vi "Write Scheduled.vi"(1 "scheduled time":timestamp, 2 "element":bool) -> (5 "actual time":timestamp, 7 "channel":T1, 8 "previous element":bool)   [LabVIEW 2020, in "Tag-bool.lvlib"]
doc: "Writes a value to a Tag channel at the scheduled time."
uses:
  <extravilib>/ChannelInstances/Tag-bool.lvlib
  <extravilib>/ChannelInstances/Tag-bool/))Channel.ctl
  <extravilib>/ChannelInstances/Tag-bool/Write With Abort.vi
  <extravilib>/ChannelInstances/Tag-bool/Endpoint.vi
  <resource>/ChannelSupport/_ChannelSupport/_ChannelSupport.lvlib
  <resource>/ChannelSupport/_ChannelSupport/GetErrors/FpgaChannelWireNotSupported.xnode
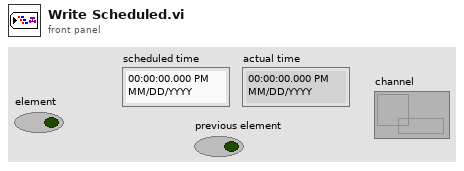
[diagram p1: front panel]
types:
  T1 = typedef "Tag-bool.lvlib/))Channel.ctl" = refnum<queue>
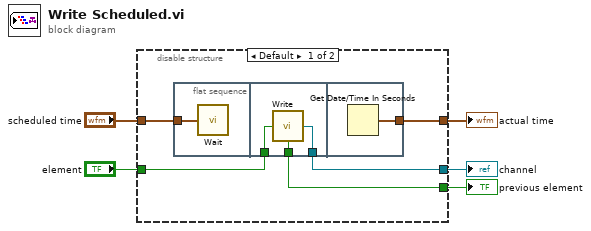
[diagram p0: block diagram]
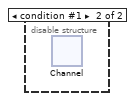
[diagram p2: hidden frame]
diagram:
  n1 = disable-structure shown="Default" {
    disable-tunnel: "scheduled time" -> [w10 _]
    disable-tunnel: [w9 _] -> w4
    disable-tunnel: "element" -> [w8 _]
    disable-tunnel: [w7 _] -> w2
    disable-tunnel: [w6 _] -> w1
    frame condition #0 (active) {
      n2 = flat-sequence {
        tunnel: w10 -> [w11]
        tunnel: w8 -> [w14]
        tunnel: [w13] -> w7
        tunnel: [w12] -> w6
        tunnel: [w15] -> w9
        frame #0 {
          n3 = call <resource>:"Wait.vi"("desired time"=w11) -> ()  [unwired: 2 out]
        }
        frame #1 {
          n4 = call <extravilib>:"Write.vi"("element"=w14) -> ("previous element"=w12:bool, "channel"=w13:T1)
        }
        frame #2 {
          n5 = Get Date/Time In Seconds() -> (seconds since 1Jan1904=w15:timestamp)
        }
      }
    }
    frame condition #1 {
      n6 = xnode "Channel"() -> ()
    }
  }
  "channel" <- w2
  "actual time" <- w4
  "previous element" <- w1
